vi "Set Data Name.vi"(8 "错误输入":errorcluster, 9 "Data Name":string, 10 "Data":variant) -> (0 "错误输出":errorcluster, 2 "Renamed Data":variant)   [LabVIEW 2012, in "TD Tools.lvlib"]
uses:
  TD Tools.lvlib
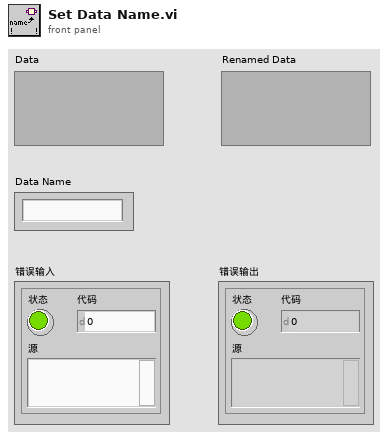
[diagram p1: front panel]
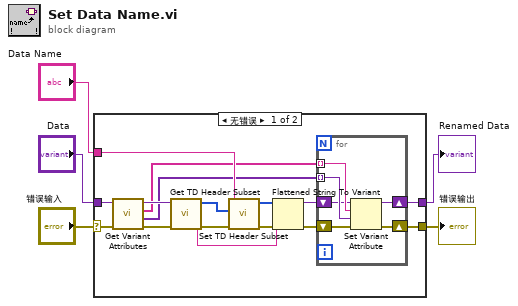
[diagram p0: block diagram]
diagram:
  n1 = case shown="无错误" "错误输入" {
    selector: "错误输入" -> [w15 w28]
    tunnel: [w12 w28] -> w2
    tunnel: [w8 _] -> w1
    tunnel: "Data Name" -> [w18 _]
    tunnel: "Data" -> [w17 _]
    frame No Error {
      n2 = call "Get Variant Attributes.vi"("错误输入"=w15, "Variant"=w17) -> ("错误输出"=w14:errorcluster, "Values"=w11:variant[], "Names"=w10:string[], "dup Variant"=w16:variant)  [unwired: 6 in]
      n3 = call "Get TD Header Subset.vi"("错误输入（无错误）"=w14, "Variant"=w16) -> ("错误输出"=w7:errorcluster, "Data String"=w19:string, "Type Descriptor Head Subset"=w21:u16[])  [unwired: 7 in]
      n4 = call "Set TD Header Subset.vi"("错误输入"=w7, "Type Descriptor Head Subse"=w21, "Data Name"=w18) -> ("错误输出"=w6:errorcluster, "Type Descriptor Head Subset输出"=w20:u16[])  [unwired: 7 in]
      n5 = Flattened String To Variant(4:w6, 6:w19, 7:w20) -> (0:w13:errorcluster, 3:w9:variant)
      n6 = for {
        shift-right: [w26] -> w12
        shift-left: w13 -> [w27]
        tunnel: w11 -> [w25] mode=indexing
        tunnel: w10 -> [w24] mode=indexing
        shift-right: [w22] -> w8
        shift-left: w9 -> [w23]
        n7 = Set Variant Attribute(Variant=w23, name=w24, value=w25, error in=w27) -> (Variant out=w22:variant, error out=w26:errorcluster)  [unwired: 1 out]
      }
    }
    frame Error {
    }
  }
  "错误输出" <- w2
  "Renamed Data" <- w1
